vi "LogDiskSpace.vi"(8 "error in":errorcluster) -> (0 "error out":errorcluster)   [LabVIEW 2018, in "feGEM DataPacker.lvlib"]
uses:
  feGEM DataPacker.lvlib
  ffe29585-e50d-4f04-a334-ed30d78a8e94.vi
  ffe29585-e50d-4f04-a334-ed30d78a8e94.vi/82aba83c-864a-4344-a2aa-567469491b62.vi
  <vilib>/Utility/SystemLogging/Write to System Log.vi
panel:
  out "Free space (gb)":dbl[](array[numeric])
  out "Size (gb)":dbl[](array[numeric])
  out "Drive letter":string[](array[string])
  out "% free":dbl[](array[numeric])
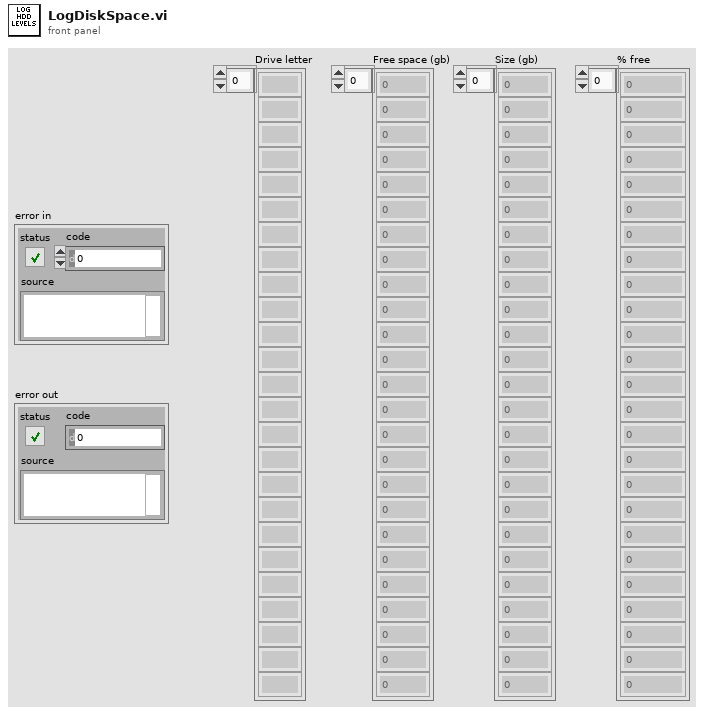
[diagram p1: front panel]
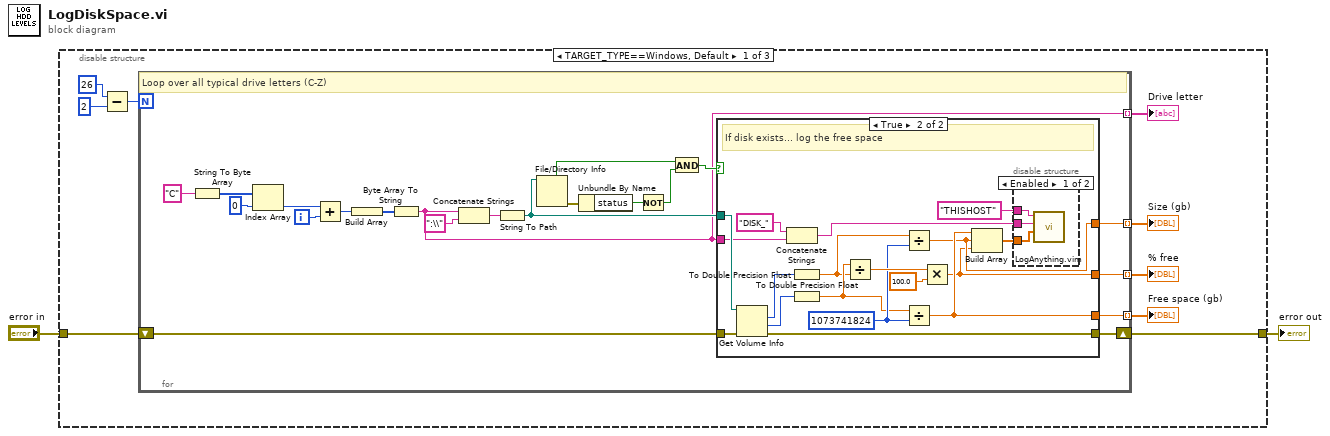
[diagram p0: block diagram]
diagram:
  n1 = disable-structure shown="TARGET_TYPE==Windows, Default" {
    disable-tunnel: "error in" -> [w4 w55 w56]
    disable-tunnel: [w3 w55 w56] -> w1
    frame condition #0 (active) {
      n2 = Subtract(x=26, y=2) -> (x-y=w11:i32)
      n3 = for {
        N: w11 -> [_]
        tunnel: [w23] -> w10 mode=indexing
        tunnel: [w14] -> w9 mode=indexing
        tunnel: [w16] -> w8 mode=indexing
        tunnel: [w15] -> w7 mode=indexing
        shift-right: [w12] -> w3
        shift-left: w4 -> [w13]
        i -> [w31]
        # "Loop over all typical drive letters (C-Z)"
        n4 = String To Byte Array(string="C") -> (unsigned byte array=w30:u8[])
        n5 = Index Array(array=w30, index=0) -> (element=w28:u8)
        n6 = Add(x=w28, y=w31) -> (x+y=w27:i32)
        n7 = Build Array(w27) -> (w26:i32[])
        n8 = Byte Array To String(unsigned byte array=w26) -> (string=w14:string)
        n9 = Concatenate Strings(w14, ":\\" ("string")) -> (w24:string)
        n10 = String To Path(string=w24) -> (path=w20:path)
        n11 = File/Directory Info(path=w20) -> (directory=w19:bool, error out=w22:errorcluster)  [unwired: 1 in, 5 out]
        n12 = Unbundle By Name(w22) -> ("status"=w21:bool)
        n13 = Not(x=w21) -> (.not. x?=w18:bool)
        n14 = And(x=w19, y=w18) -> (x .and. y?=w17:bool)
        n15 = case shown="True" w17 {
          tunnel: w20 -> [_ w51]
          tunnel: [_ w39] -> w23
          tunnel: [_ w40] -> w16
          tunnel: [_ w41] -> w15
          tunnel: w14 -> [_ w43]
          tunnel: w13 -> [w33 w37]
          tunnel: [w33 w36] -> w12
          frame False {
          }
          frame True {
            w46 = i64 1073741824 ("y")
            # "If disk exists... log the free space"
            n16 = Get Volume Info(8:w37, 11:w51) -> (0:w36:errorcluster, 1:w47:i64, 2:w48:i64)  [unwired: 3 out]
            n17 = Concatenate Strings("DISK_", w43) -> (w42:string)
            n18 = To Double Precision Float(number=w48) -> (double precision float=w34:dbl)
            n19 = To Double Precision Float(number=w47) -> (double precision float=w35:dbl)
            n20 = Divide(x=w35, y=w34) -> (x/y=w50:dbl)
            n21 = Divide(x=w34, y=w46) -> (x/y=w40:dbl)
            n22 = Divide(x=w35, y=w46) -> (x/y=w41:dbl)
            n23 = Multiply(x=w50, y=100.0) -> (x*y=w39:dbl)
            n24 = Build Array(w41, w40, w39) -> (w38:dbl[])
            n25 = disable-structure shown="Enabled" {
              disable-tunnel: "THISHOST" ("Category") -> [w54 _]
              disable-tunnel: w42 -> [w53 _]
              disable-tunnel: w38 -> [w52 _]
              frame Enabled {
                n26 = call "LogAnything.vim"("Array"=w52, "Variable Name"=w53, "Category"=w54) -> ()  [unwired: 7 in, 2 out]
              }
              frame Disabled {
              }
            }
          }
        }
      }
      "% free" <- w10
      "Drive letter" <- w9
      "Size (gb)" <- w8
      "Free space (gb)" <- w7
    }
    frame condition #1 {
    }
    frame condition #2 {
    }
  }
  "error out" <- w1
